vi "TEMPGetType.vi"(8 "error in (no error)":errorcluster, 11 "Actor in":refnum<class "Actor.lvclass">) -> (0 "error out":errorcluster, 2 "Data Sample":variant, 3 "Actor out":refnum<class "Actor.lvclass">)   [LabVIEW 2015, in "PV Message Template.lvclass"]
uses:
  PV Message Template.lvclass
  <vilib>/ActorFramework/Actor/Actor.lvclass
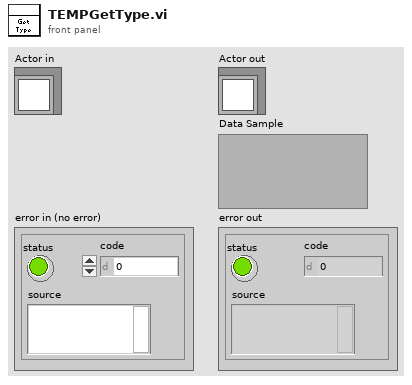
[diagram p1: front panel]
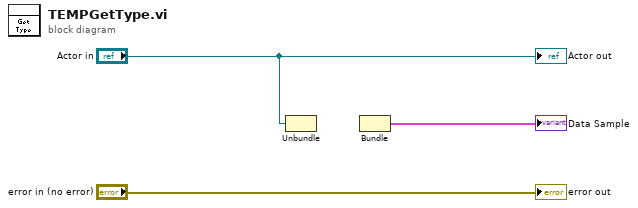
[diagram p0: block diagram]
diagram:
  n1 = Unbundle("Actor in") -> ()  [unwired: 2 out]
  n2 = Bundle() -> (→"Data Sample":cluster{void, void})  [unwired: 3 in]
  "error out" <- "error in (no error)"
  "Actor out" <- "Actor in"
